vi "RageEquipCal_Lookup.vi"(0 "Record(abs path)":path=path "C:/SynologyDrive/ RaGE Systems/Test Equipment Cal Record/Rage_TestEquipmentCal.csv", 5 "SN / Active(1=T)":string[][](array[string])=[["MY53271104", "1"], ["MY57470396", "1"], ["MY48180752", "1"]], 11 "error in (no error)":errorcluster, 12 "Use Popup Warning(T)":bool=TRUE caption="Use Popup (T)", 13 "Run Vi (T)":bool=TRUE, 14 "Use Popup Warning(T)":bool caption="Check All SN's On List (T)") -> (4 "Status Summary Out":string[][](array[string]), 6 "OK":bool=TRUE, 15 "error out":errorcluster)   [LabVIEW 2018]
uses:
  Initialize References/Sequence Globals.vi
  <vilib>/Utility/file.llb/Read Delimited Spreadsheet (string).vi
  <vilib>/Utility/file.llb/Write Delimited Spreadsheet (string).vi
panel:
  out "RecordTempPath":path
  out "tmp path":path
  out "Mfr":string="RGA21-0197"
  out "Mfr_Index":i32
  out "Remind_Index":i32
  out "Active_index":i32[](array[numeric])=[11, 13, 14]
  out "ActiveList":string[][](array[string])
  out "RecordTempPath(str)":string="C:\\SynologyDrive\\ RaGE Systems\\Test Equipment Cal Record\\Rage_TestEquipmentCal.csv"
  out "HeaderMatchNames":string[](array[string])=["Model", "Last Cal Date", "SN", "Cal Due Date", "Desc", "Asset"]
  out "Header Match?":bool=TRUE
  out "expired?":bool=TRUE
  out "warn?":bool=TRUE
  out "Now":timestamp=timestamp(3806421519 s since 1904-01-01)
  out "Warn_Date":timestamp=timestamp(3776216400 s since 1904-01-01)
  out "seconds":dbl=2592000.0
  out "Warn (days)":string="30"
  out "last_cal(date)":timestamp=timestamp(3778808400 s since 1904-01-01)
  out "next_cal(date)":timestamp=timestamp(3778808400 s since 1904-01-01)
  out "asset":string="RGA21-0197"
  out "Asset_Index":i32
  out "desc":string="SIGGEN"
  out "Desc_Index":i32=6
  out "sn":string="MY48180752"
  out "next_cal(str)":string="9/29/2023"
  out "last_cal(str)":string="9/29/2020"
  out "model":string="N5182A"
  out "SnMatch?":bool=TRUE
  out "data_rows":string[][](array[string])=[["", "", "Anritsu", "37369C", "Yes", "", "VNA", "REPAIR(LOW)?", "", "", "E15539", "1/1/2001", "1/1/2001", "", "N/A", "N/A"], ["", "12989", "AstroAI", "DM6000AR", "Yes", "", "DMM", "LOWELL", "RaGE Systems", "", "2125220590", "1/1/2001", "1/1/2001", "", "N/A", "N/A"], ["", "12990", "AstroAI", "DM6000AR", "Yes", "", "DMM", "LOWELL", "RaGE Systems", "", "2125219987", "1/1/2001", "1/1/2001", "", "N/A", "N/A"], ["RGA20-0121", "", "Keithly", "2000", "Yes", "LAB-DC", "DMM", "LOWELL", "RaGE Systems", "Purchased", "727501", "1/1/2001", "1/1/2001", "", "N/A", "N/A"], ["RGA20-0123", "", "Keithly", "2000", "Yes", "LAB-DC", "DMM", "LOWELL", "RaGE Systems", "Purchased", "822794", "1/1/2001", "1/1/2001", "", "N/A", "N/A"], ["", "12937", "Keithly", "2000", "Yes", "Keithley 2000 Multimeters ", "DMM", "LOWELL", "RaGE Systems", "", "735571", "9/25/2019", "9/25/2020", "", "N/A", "N/A"], ["", "13071", "Keithly", "2700", "No", "LAB-DC", "DAQ", "LOWELL", "RaGE Systems", "", "", "Cal Not Required", "Cal Not Required", "", "N/A", "N/A"], ["RGA19-0071", "12928", "Keysight", "E5052A", "Yes", "LAB-RF", "Signal Source Analyzer", "LOWELL", "RaGE Systems (PRF)", "PRF", "MY44200746", "1/1/2001", "1/1/2001", "", "N/A", "N/A"], ["RGA19-0078", "12944", "Keysight", "8720ES", "Yes", "LAB-RF", "VNA", "LOWELL", "RaGE Systems", "Ks MVO -ebay", "US39173304", "8/28/2017", "8/28/2018", "F-Support  ", "N/A", "N/A"], ["RGA20-0130", "", "Keysight", "U2022XA", "Yes", "LAB-RF", "Power Meter", "WAM-PROD", "RaGE Systems", "Keysight", "MY58240013", "6/19/2018", "6/19/2020", "F-Support  ", "N/A", "TBD"], ["RGA20-0150", "", "Keysight", "N4692A", "Yes", "LAB-RF", "E-Cal Module", "WAM-PROD", "RaGE Systems", "Purchased", "MY62230410", "9/18/2019", "9/18/2021", "T", "N/A", "N/A"], ["RGA21-0195", "", "Keysight", "N5173B", "Yes", "LAB-RF", "Signal Generator", "WAM ATE-2", "RaGE Systems", "Purchased", "MY53271104", "11/6/2019", "11/6/2022", "T", "N/A", "1/19/2020"], ["RGA21-0224", "", "Keysight", "N5232B ", "Yes", "LAB-RF", "PNA", "WAM ATE-2", "RaGE Systems", "Purchased", "MY52221531", "2/20/2020", "2/20/2022", "T", "N/A", "N/A"], ["RGA21-0226", "", "Keysight", "N9010B", "No", "LAB-RF", "Spectrum Analyzer", "WAM ATE-2", "RaGE Systems", "Purchased", "MY57470396", "9/30/2023", "9/30/2025", "T", "N/A", "4/10/2025"], ["RGA21-0197", "12943", "Keysight", "N5182A", "Yes", "LAB-RF", "SIGGEN", "LOWELL", "RaGE Systems", "Purchased", "MY48180752", "9/29/2020", "9/29/2023", "T", "11/30/2024", "11/30/2023"], ["RGA21-0196", "", "Keysight", "N9010B", "Yes", "LAB-RF", "Spectrum Analyzer", "KS REPAIR", "RaGE Systems", "Purchased", "MY57110230", "11/3/2021", "11/3/2023", "T", "7/23/2024", "7/23/2024"], ["RGA21-0223", "12941", "Keysight", "N9020A", "Yes", "LAB-RF", "Spectrum Analyzer", "LOWELL", "Interlligent (Rental)", "Rent2Own", "MY49100234", "4/8/2021", "4/8/2023", "T", "N/A", "N/A"], ["RGA21-0222", "", "Keysight", "N5173B", "Yes", "LAB-RF", "SIGGEN", "WAM ATE-1", "RaGE Systems", "Purchased", "MY53270534 ", "6/12/2020", "6/12/2023", "T", "7/19/2020", "1/19/2021"], ["RGA21-0225", "", "Keysight", "N5232A", "Yes", "LAB-RF", "PNA", "WAM ATE-1", "RaGE Systems", "Purchased", "US52120122", "4/21/2021", "4/21/2023", "T", "6/6/2019", "6/8/2019"], ["RGA20-0149", "12945", "Keysight", "N5224B", "Yes", "LAB-RF", "PNA-X", "NBPT", "RaGE Systems", "Purchased", "MY55441806", "11/19/2019", "11/19/2021", "T", "2/11/2026", "2/11/2026"], ["N/A", "", "Keysight", "E4447A", "Yes", "LAB-RF", "Spectrum Analyzer", "WAM ATE-1", "LEIDOS", "Loaner", "MY9420095", "1/1/2001", "1/1/2001", "F  ", "N/A", "N/A"], ["RGA18-0064", "12942", "Keysight / Agilent", "E4433B", "Yes", "LAB-RF", "Signal Generator", "LOWELL", "RaGE Systems", "Ebay", "US40051660", "TBD", "TBD", "F-Support", "", ""], ["RGA18-0006", "12935", "Keysight / Agilent", "34401A", "Yes", "LAB-DC", "DMM", "LOWELL", "RaGE Systems", "Ebay", "MY44006486", "TBD", "TBD", "F-Support", "", ""], ["RGA18-0065", "12914", "Keysight / HP", "E4405B", "Yes", "LAB-RF", "Spectrum Analyzer", "LOWELL", "RaGE Systems", "Ebay", "US39440417", "TBD", "TBD", "F-Support", "", ""], ["RGA19-0072", "", "MINI - CIRCUITS", "PWR-6GHS", "Yes", "LAB-RF", "Power Meter", "LOWELL", "RaGE Systems", "PRF", "11807080018", "TBD", "TBD", "", "", ""], ["RGA19-0088", "", "National Instruments", "USB-TC01", "No", "LAB-Test", "Thermocouple", "LOWELL", "RaGE Systems", "Purchased", "N/A", "N/A", "N/A", "", "", ""], ["RGA18-0057", "13072", "Omega", "TCIC", "No", "LAB-Test", "Thermocouple", "LOWELL", "RaGE Systems", "Purchased", "N/A", "N/A", "N/A", "", "", ""], ["RGA20-0104", "", "Vaunix", "LPS-802", "No", "LAB-Test", "Vaunix Lab Brick LPS-802 4 – 8 GHz USB Programmable Phase Shifter", "LOWELL", "RaGE Systems", "Purchased", "N/A", "N/A", "N/A", "", "", ""], ["RGA20-0105", "12900", "Vaunix", "LDA-602", "No", "LAB-Test", "Vaunix Lab Brick Digital Attenuator LDA-602", "LOWELL", "RaGE Systems", "Purchased", "N/A", "N/A", "N/A", "", "", ""]]
  out "SN_Index":i32=10
  out "Model_Index":i32=3
  out "NextCal_Index":i32=12
  out "LastCal_Index":i32=11
  out "Record(ary)":string[][](array[string])=[["Asset", "Security Label Number", "Manufacturer", "Model", "Calibration Required (Yes/No)", "Type", "Desc", "Location or User", "Owner / Loan", "Provided By", "SN", "Last Cal Date", "Cal Due Date", "Keysight Asseted", "Keysight Cal Entitlement Expires", "Keysight Warranty Expires"], ["", "", "Anritsu", "37369C", "Yes", "", "VNA", "REPAIR(LOW)?", "", "", "E15539", "1/1/2001", "1/1/2001", "", "N/A", "N/A"], ["", "12989", "AstroAI", "DM6000AR", "Yes", "", "DMM", "LOWELL", "RaGE Systems", "", "2125220590", "1/1/2001", "1/1/2001", "", "N/A", "N/A"], ["", "12990", "AstroAI", "DM6000AR", "Yes", "", "DMM", "LOWELL", "RaGE Systems", "", "2125219987", "1/1/2001", "1/1/2001", "", "N/A", "N/A"], ["RGA20-0121", "", "Keithly", "2000", "Yes", "LAB-DC", "DMM", "LOWELL", "RaGE Systems", "Purchased", "727501", "1/1/2001", "1/1/2001", "", "N/A", "N/A"], ["RGA20-0123", "", "Keithly", "2000", "Yes", "LAB-DC", "DMM", "LOWELL", "RaGE Systems", "Purchased", "822794", "1/1/2001", "1/1/2001", "", "N/A", "N/A"], ["", "12937", "Keithly", "2000", "Yes", "Keithley 2000 Multimeters ", "DMM", "LOWELL", "RaGE Systems", "", "735571", "9/25/2019", "9/25/2020", "", "N/A", "N/A"], ["", "13071", "Keithly", "2700", "No", "LAB-DC", "DAQ", "LOWELL", "RaGE Systems", "", "", "Cal Not Required", "Cal Not Required", "", "N/A", "N/A"], ["RGA19-0071", "12928", "Keysight", "E5052A", "Yes", "LAB-RF", "Signal Source Analyzer", "LOWELL", "RaGE Systems (PRF)", "PRF", "MY44200746", "1/1/2001", "1/1/2001", "", "N/A", "N/A"], ["RGA19-0078", "12944", "Keysight", "8720ES", "Yes", "LAB-RF", "VNA", "LOWELL", "RaGE Systems", "Ks MVO -ebay", "US39173304", "8/28/2017", "8/28/2018", "F-Support  ", "N/A", "N/A"], ["RGA20-0130", "", "Keysight", "U2022XA", "Yes", "LAB-RF", "Power Meter", "WAM-PROD", "RaGE Systems", "Keysight", "MY58240013", "6/19/2018", "6/19/2020", "F-Support  ", "N/A", "TBD"], ["RGA20-0150", "", "Keysight", "N4692A", "Yes", "LAB-RF", "E-Cal Module", "WAM-PROD", "RaGE Systems", "Purchased", "MY62230410", "9/18/2019", "9/18/2021", "T", "N/A", "N/A"], ["RGA21-0195", "", "Keysight", "N5173B", "Yes", "LAB-RF", "Signal Generator", "WAM ATE-2", "RaGE Systems", "Purchased", "MY53271104", "11/6/2019", "11/6/2022", "T", "N/A", "1/19/2020"], ["RGA21-0224", "", "Keysight", "N5232B ", "Yes", "LAB-RF", "PNA", "WAM ATE-2", "RaGE Systems", "Purchased", "MY52221531", "2/20/2020", "2/20/2022", "T", "N/A", "N/A"], ["RGA21-0226", "", "Keysight", "N9010B", "No", "LAB-RF", "Spectrum Analyzer", "WAM ATE-2", "RaGE Systems", "Purchased", "MY57470396", "9/30/2023", "9/30/2025", "T", "N/A", "4/10/2025"], ["RGA21-0197", "12943", "Keysight", "N5182A", "Yes", "LAB-RF", "SIGGEN", "LOWELL", "RaGE Systems", "Purchased", "MY48180752", "9/29/2020", "9/29/2023", "T", "11/30/2024", "11/30/2023"], ["RGA21-0196", "", "Keysight", "N9010B", "Yes", "LAB-RF", "Spectrum Analyzer", "KS REPAIR", "RaGE Systems", "Purchased", "MY57110230", "11/3/2021", "11/3/2023", "T", "7/23/2024", "7/23/2024"], ["RGA21-0223", "12941", "Keysight", "N9020A", "Yes", "LAB-RF", "Spectrum Analyzer", "LOWELL", "Interlligent (Rental)", "Rent2Own", "MY49100234", "4/8/2021", "4/8/2023", "T", "N/A", "N/A"], ["RGA21-0222", "", "Keysight", "N5173B", "Yes", "LAB-RF", "SIGGEN", "WAM ATE-1", "RaGE Systems", "Purchased", "MY53270534 ", "6/12/2020", "6/12/2023", "T", "7/19/2020", "1/19/2021"], ["RGA21-0225", "", "Keysight", "N5232A", "Yes", "LAB-RF", "PNA", "WAM ATE-1", "RaGE Systems", "Purchased", "US52120122", "4/21/2021", "4/21/2023", "T", "6/6/2019", "6/8/2019"], ["RGA20-0149", "12945", "Keysight", "N5224B", "Yes", "LAB-RF", "PNA-X", "NBPT", "RaGE Systems", "Purchased", "MY55441806", "11/19/2019", "11/19/2021", "T", "2/11/2026", "2/11/2026"], ["N/A", "", "Keysight", "E4447A", "Yes", "LAB-RF", "Spectrum Analyzer", "WAM ATE-1", "LEIDOS", "Loaner", "MY9420095", "1/1/2001", "1/1/2001", "F  ", "N/A", "N/A"], ["RGA18-0064", "12942", "Keysight / Agilent", "E4433B", "Yes", "LAB-RF", "Signal Generator", "LOWELL", "RaGE Systems", "Ebay", "US40051660", "TBD", "TBD", "F-Support", "", ""], ["RGA18-0006", "12935", "Keysight / Agilent", "34401A", "Yes", "LAB-DC", "DMM", "LOWELL", "RaGE Systems", "Ebay", "MY44006486", "TBD", "TBD", "F-Support", "", ""], ["RGA18-0065", "12914", "Keysight / HP", "E4405B", "Yes", "LAB-RF", "Spectrum Analyzer", "LOWELL", "RaGE Systems", "Ebay", "US39440417", "TBD", "TBD", "F-Support", "", ""], ["RGA19-0072", "", "MINI - CIRCUITS", "PWR-6GHS", "Yes", "LAB-RF", "Power Meter", "LOWELL", "RaGE Systems", "PRF", "11807080018", "TBD", "TBD", "", "", ""], ["RGA19-0088", "", "National Instruments", "USB-TC01", "No", "LAB-Test", "Thermocouple", "LOWELL", "RaGE Systems", "Purchased", "N/A", "N/A", "N/A", "", "", ""], ["RGA18-0057", "13072", "Omega", "TCIC", "No", "LAB-Test", "Thermocouple", "LOWELL", "RaGE Systems", "Purchased", "N/A", "N/A", "N/A", "", "", ""], ["RGA20-0104", "", "Vaunix", "LPS-802", "No", "LAB-Test", "Vaunix Lab Brick LPS-802 4 – 8 GHz USB Programmable Phase Shifter", "LOWELL", "RaGE Systems", "Purchased", "N/A", "N/A", "N/A", "", "", ""], ["RGA20-0105", "12900", "Vaunix", "LDA-602", "No", "LAB-Test", "Vaunix Lab Brick Digital Attenuator LDA-602", "LOWELL", "RaGE Systems", "Purchased", "N/A", "N/A", "N/A", "", "", ""]]
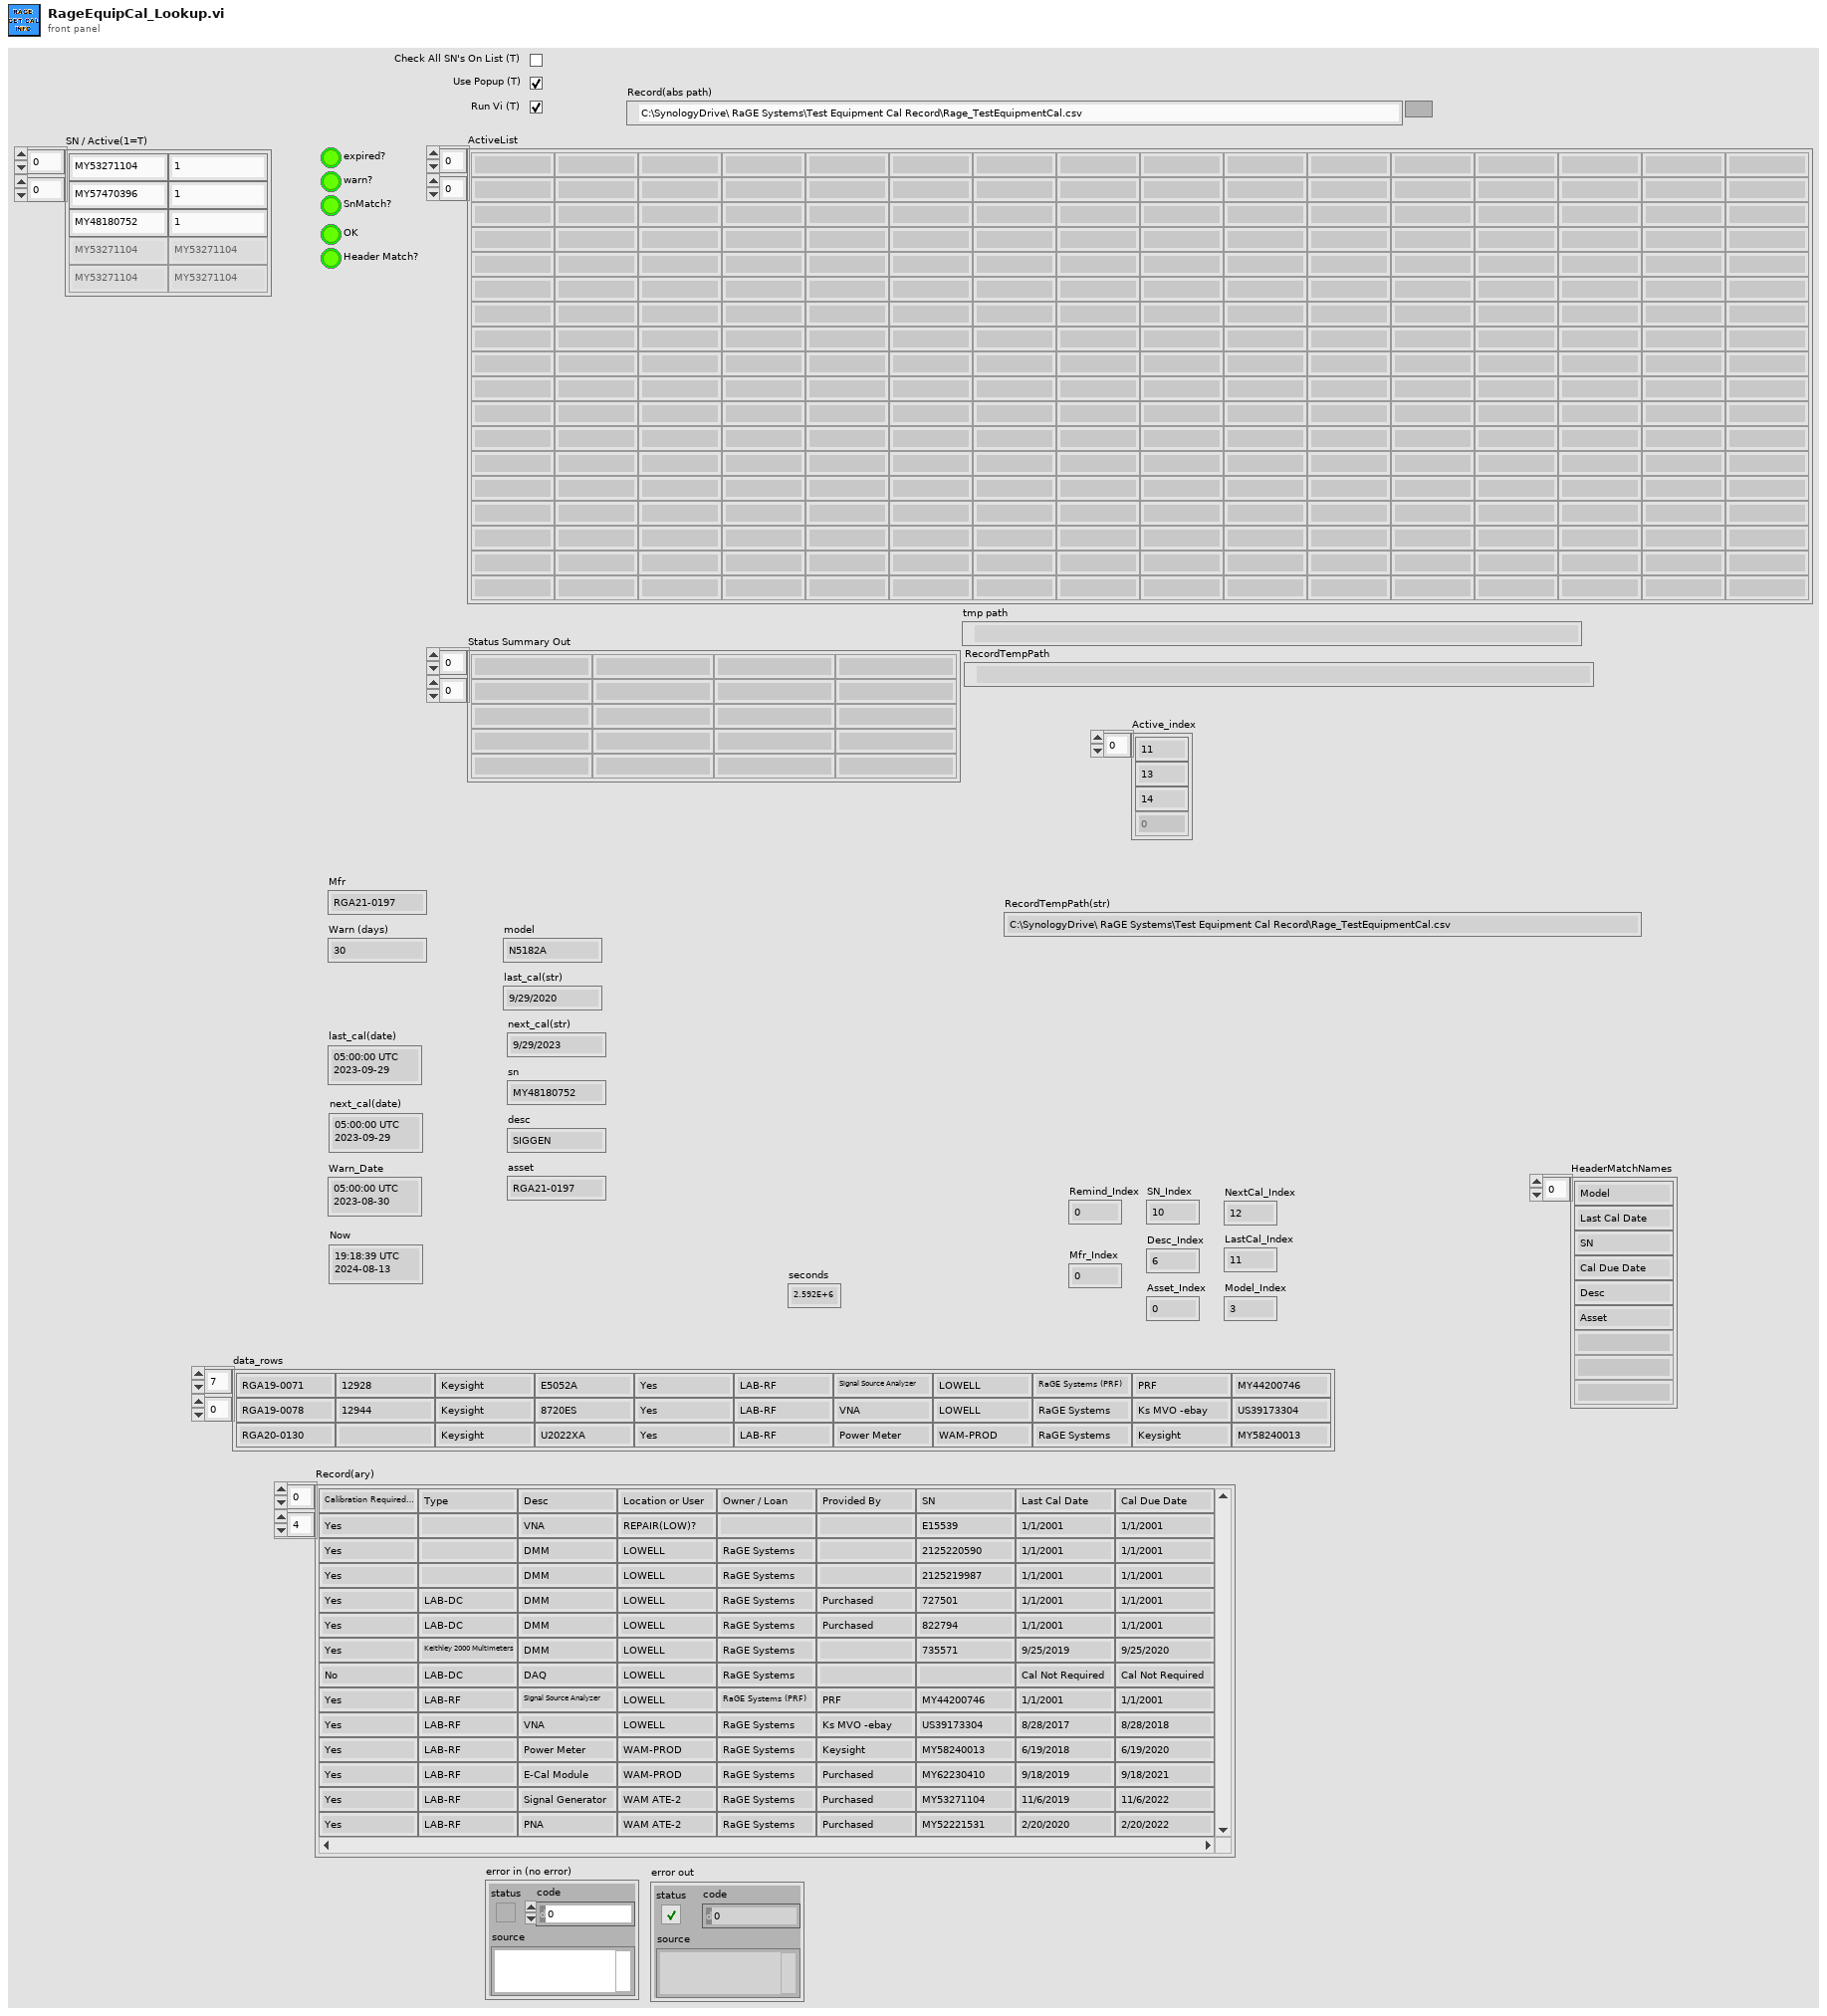
[diagram p1: front panel]
types:
  T1 = enum16{"Left Button", "Center Button", "Right Button", "Window Close"}
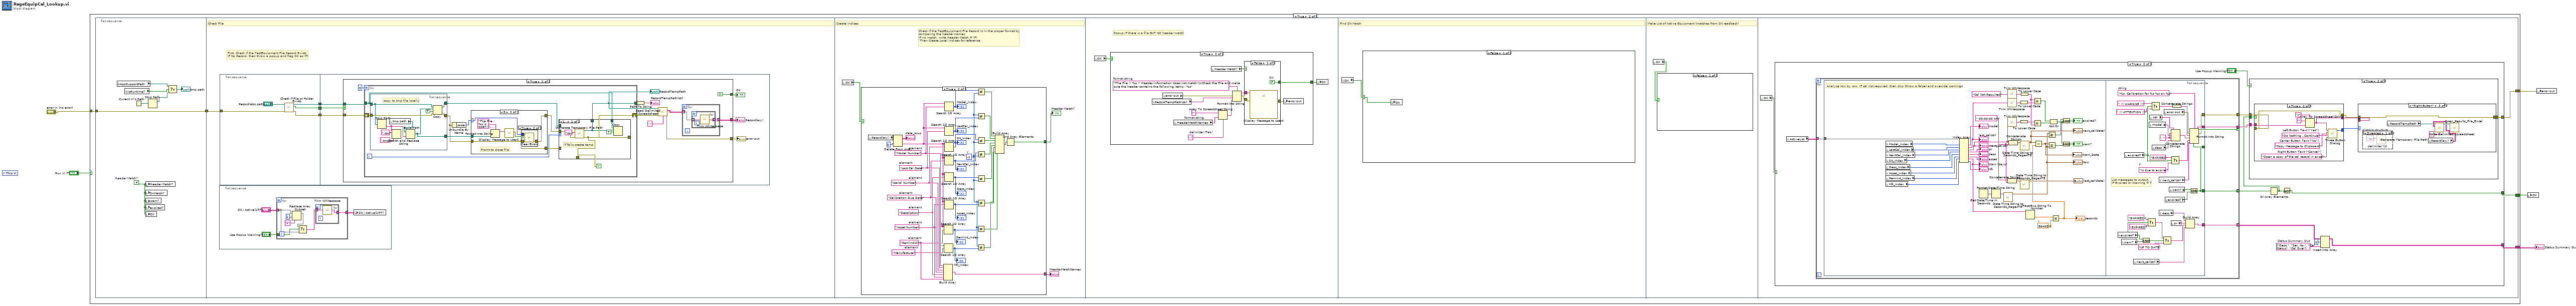
[diagram p0: block diagram]
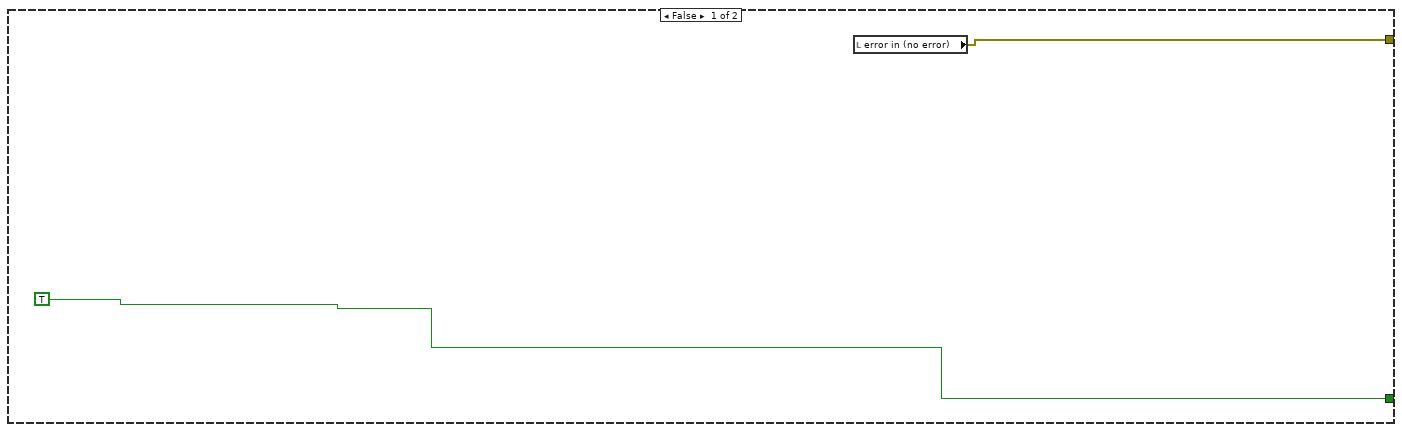
[diagram p2: hidden frame]
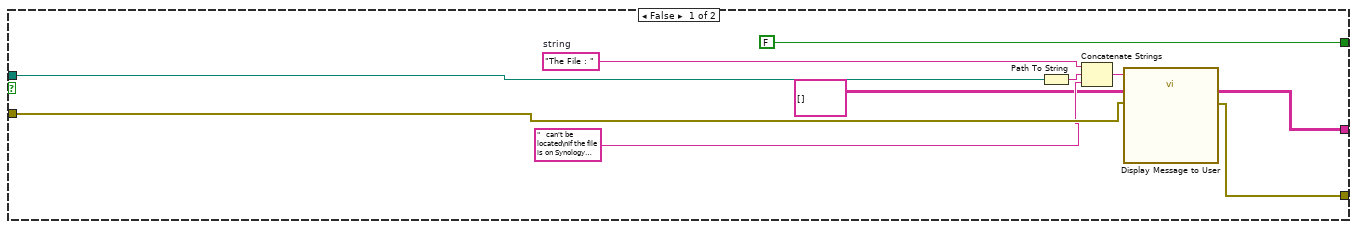
[diagram p3: hidden frame]
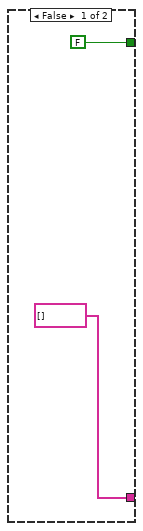
[diagram p7: hidden frame]
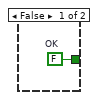
[diagram p8: hidden frame]
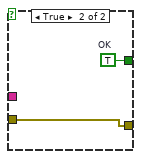
[diagram p9: hidden frame]
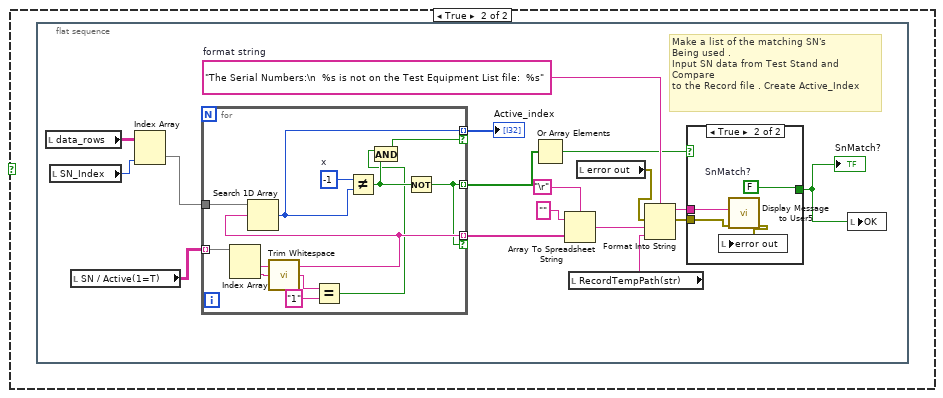
[diagram p10: hidden frame]
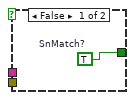
[diagram p11: hidden frame]
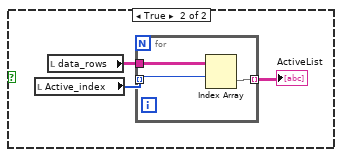
[diagram p12: hidden frame]
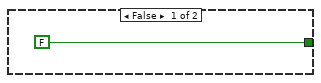
[diagram p13: hidden frame]
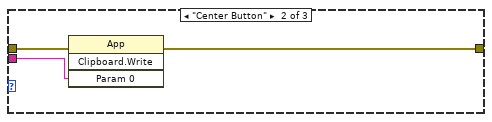
[diagram p16: hidden frame]
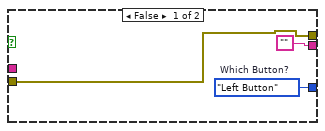
[diagram p18: hidden frame]
diagram:
  n1 = control-ref of="This VI"() -> ()  [unwired: 1 out]
  n2 = case shown="True" "Run Vi (T)" {
    tunnel: "error in (no error)" -> [_ w12]
    tunnel: [w7 w11] -> w4
    tunnel: [TRUE w10] -> w2
    tunnel: [_ w9] -> w1
    frame False {
      n3 = local read "error in (no error)"() -> (w7:errorcluster)
    }
    frame True {
      n4 = flat-sequence {
        tunnel: w12 -> [w19]
        tunnel: [w19] -> w8
        tunnel: w8 -> [w20]
        tunnel: [w218] -> w11
        tunnel: [w217] -> w10
        tunnel: [w216] -> w9
        frame #0 {
          w18 = FALSE  # Header Match?
          n5 = global read "Sequence Globals.vi" "AppSupportPath"() -> (w16:path)
          n6 = global read "Sequence Globals.vi" "IsRuntime?"() -> (w17:bool)
          n7 = Current VI's Path() -> (path=w15:path)
          n8 = local write "Header Match?"(w18) -> ()
          n9 = local write "SnMatch?"(w18) -> ()
          n10 = local write "warn?"(w18) -> ()
          n11 = local write "expired?"(w18) -> ()
          n12 = local write "OK"(w18) -> ()
          n13 = Strip Path(path=w15) -> (stripped path=w14:path)  [unwired: 1 out]
          n14 = Select(t=w16, s=w17, f=w14) -> (s? t:f=→"tmp path":path)
        }
        frame #1 {
          # "First, Check If the TestEquipment File Record Exists\nIF No Record, then throw a popup and flag OK as (F)"
          # "Check File"
          n15 = flat-sequence {
            frame #0 {
              n16 = for {
                tunnel: "SN / Active(1=T)" -> [w30] mode=indexing
                tunnel: [w33] -> w25 mode=indexing
                tunnel: "Use Popup Warning(T)" -> [w27]
                n17 = Replace Array Subset(array=w30, new element="1" ("new element/subarray"), index=1) -> (w28:string[])
                n18 = Select(t=w28, s=w27, f=w30) -> (s? t:f=w29:string[])
                n19 = for {
                  tunnel: w29 -> [w35] mode=indexing
                  tunnel: [w34] -> w33 mode=indexing
                  n20 = call <vilib>:"Trim Whitespace.vi"("string"=w35) -> ("trimmed string"=w34:string)  [unwired: 1 in]
                }
              }
              n21 = local write "SN / Active(1=T)"(w25) -> ()
            }
          }
          n22 = flat-sequence {
            tunnel: [w39] -> w23
            tunnel: [w40] -> w22
            tunnel: [w38] -> w21
            tunnel: w20 -> [w37]
            tunnel: w23 -> [w46]
            tunnel: w22 -> [w45]
            tunnel: w21 -> [w44]
            frame #0 {
              n23 = call <vilib>:"Check if File or Folder Exists.vi"("error in (no error)"=w37, "path"="Record(abs path)") -> ("error out"=w40:errorcluster, "file or folder exists?"=w39:bool, "dup path"=w38:path)  [unwired: 7 in]
            }
            frame #1 {
              n24 = case shown="True" w46 {
                tunnel: w45 -> [w50 w62]
                tunnel: w44 -> [w55 w63]
                tunnel: [FALSE TRUE] -> w43
                tunnel: [w49 w60] -> w42
                tunnel: [string[][] [] w64] -> w41
                frame False {
                  w53 = "The File : "  # string
                  n25 = Path To String(path=w55) -> (string=w54:string)
                  n26 = Concatenate Strings(w53, w54, "   can't be located\nIf the file is on Synology Drive check the connection to the server" ("string")) -> (w52:string)
                  n27 = call "Display Message to User"("error in (no error)"=w50, "Message"=w52) -> ("error out"=w49:errorcluster)  [unwired: 8 in, 1 out]
                }
                frame True {
                  n28 = for {
                    N: 3 -> [_]
                    shift-right: [w71] -> w58
                    shift-left: w62 -> [w78]
                    tunnel: w63 -> [w67]
                    tunnel: [w72] -> w57
                    i -> [w75]
                    stop <- w69 continue-if-true
                    n29 = flat-sequence {
                      tunnel: w67 -> [w102]
                      tunnel: w78 -> [w108]
                      tunnel: [w107] -> w70
                      tunnel: [w106] -> w73
                      tunnel: [w100] -> w76
                      frame #0 {
                        # "copy to tmp file locally"
                        n30 = Strip Path(path=w102) -> (name=w101:string)  [unwired: 1 out]
                        n31 = local read "tmp path"() -> (w103:path)
                        n32 = Search and Replace String(input string=w101, search string=".csv", replace string=".tmp" ("replace string (\"\")")) -> ()  [unwired: 5 in, 4 out]
                        n33 = Build Path(base path=w103, name or relative path=w101) -> (appended path=w100:path)
                        n34 = Copy(8:w108, 9:TRUE ("overwrite (F)"), 10:w100, 11:w102) -> (0:w107:errorcluster, 3:w106:path)  [unwired: 1 in, 1 out]
                      }
                    }
                    n35 = Unbundle By Name(w70) -> ("code"=w77:i32)
                    n36 = case shown="5" w77 {
                      selector: w77 -> [_ w91]
                      tunnel: [w88 w93] -> w74
                      tunnel: w70 -> [w88 w89]
                      tunnel: w76 -> [_ w92]
                      tunnel: [w88 w89] -> w68
                      frame 0, Default {
                      }
                      frame 5 {
                        # "Promt to close file"
                        n37 = Format Into String(format string="The File : %s is open!! \nClose the file and press OK to continue", w92) -> (resulting string=w94:string)  [unwired: 2 in, 1 out]
                        n38 = call "Display Message to User2"("Message"=w94) -> ("OK"=w90:bool)  [unwired: 9 in, 1 out]
                        n39 = case shown="True" w90 {
                          tunnel: [w96 w99] -> w93
                          tunnel: w91 -> [_ w98]
                          tunnel: w89 -> [w96 w97]
                          frame False {
                          }
                          frame True {
                            n40 = call <vilib>:"Clear Errors.vi"("error in (no error)"=w97, "specific error code to clear (0: all)"=w98) -> ("error out"=w99:errorcluster)  [unwired: 4 in, 1 out]
                          }
                        }
                      }
                    }
                    n41 = case shown="2.." w75 {
                      tunnel: w74 -> [w80 w87]
                      tunnel: w73 -> [w81 _]
                      tunnel: [w81 w85] -> w72
                      tunnel: [w80 w86] -> w71
                      tunnel: [w79 w86] -> w69
                      tunnel: w68 -> [w79 _]
                      tunnel: w67 -> [_ w84]
                      frame 0, Default {
                      }
                      frame 2.. {
                        # "If fails create temp"
                        n42 = call <vilib>:"Generate Temporary File Path.vi"("error in (no error)"=w87, "Temporary File Extension (tmp)"="csv") -> ("error out"=w86:errorcluster, "Unique Temporary File Path"=w85:path)  [unwired: 8 in]
                        n43 = Copy(9:TRUE ("overwrite (F)"), 10:w85, 11:w84) -> ()  [unwired: 2 in, 3 out]
                      }
                    }
                  }
                  "RecordTempPath" <- w57
                  n44 = Path To String(path=w57) -> (string=→"RecordTempPath(str)":string)
                  n45 = call-poly <vilib>:"Read Delimited Spreadsheet.vi"("file path (dialog if empty)"=w57, "error in (no error)"=w58, "delimiter (\\t)"="," ("delimiter (\\t)")) -> ("all rows"=w61:string[][], "error out"=w60:errorcluster)  [unwired: 7 in, 4 out]
                  n46 = for {
                    tunnel: w61 -> [w111] mode=indexing
                    tunnel: [w110] -> w64 mode=indexing
                    n47 = for {
                      tunnel: w111 -> [w113] mode=indexing
                      tunnel: [w112] -> w110 mode=indexing
                      n48 = call <vilib>:"Trim Whitespace.vi"("string"=w113) -> ("trimmed string"=w112:string)  [unwired: 1 in]
                    }
                  }
                }
              }
              "OK" <- w43
              "error out" <- w42
              "Record(ary)" <- w41
            }
          }
        }
        frame #2 {
          # "Check If the TestEquipment File Record Is in the proper format by\ncomparing the header names.\nIF no match, write Header Match = (F)\n Then Create Local indices for reference"
          # "Create indices"
          n49 = local read "OK"() -> (w114:bool)
          n50 = case shown="True" w114 {
            tunnel: [string[] [] w129] -> w116
            tunnel: [FALSE w127] -> w115
            frame False {
            }
            frame True {
              w119 = "Manufacturer"  # element
              w125 = "Remind(d)"  # element
              w130 = "Asset Number"  # element
              w131 = "Description"  # element
              w121 = -1  # y
              w133 = "Serial Number"  # element
              w135 = "Model Number"  # element
              w132 = "Calibration Due Date"  # element
              w134 = "Last Cal Date"  # element
              n51 = local read "Record(ary)"() -> (w150:string[][])
              n52 = Delete From Array(array=w150, index (row)=0) -> (deleted portion=w120:string[], array with subset deleted=→"data_rows":string[][])  [unwired: 2 in]
              n53 = Build Array(w135, w134, w133, w132, w131, w130, w125) -> (w129:string[])
              n54 = Search 1D Array(1D array=w120, element=w125) -> (index of element=w126:i32)  [unwired: 1 in]
              "Remind_Index" <- w126
              n55 = Search 1D Array(1D array=w120, element=w119) -> (index of element=w123:i32)  [unwired: 1 in]
              "Mfr_Index" <- w123
              n56 = Search 1D Array(1D array=w120, element=w135) -> (index of element=w147:i32)  [unwired: 1 in]
              "Model_Index" <- w147
              n57 = Search 1D Array(1D array=w120, element=w134) -> (index of element=w146:i32)  [unwired: 1 in]
              "LastCal_Index" <- w146
              n58 = Search 1D Array(1D array=w120, element=w133) -> (index of element=w145:i32)  [unwired: 1 in]
              "SN_Index" <- w145
              n59 = Search 1D Array(1D array=w120, element=w132) -> (index of element=w144:i32)  [unwired: 1 in]
              "NextCal_Index" <- w144
              n60 = Search 1D Array(1D array=w120, element=w131) -> (index of element=w143:i32)  [unwired: 1 in]
              "Desc_Index" <- w143
              n61 = Search 1D Array(1D array=w120, element=w130) -> (index of element=w142:i32)  [unwired: 1 in]
              "Asset_Index" <- w142
              n62 = Not Equal?(x=w121, y=w126) -> (x != y?=w124:bool)
              n63 = Not Equal?(x=w121, y=w123) -> (x != y?=w122:bool)
              n64 = Not Equal?(x=w147, y=w121) -> (x != y?=w141:bool)
              n65 = Not Equal?(x=w121, y=w146) -> (x != y?=w140:bool)
              n66 = Not Equal?(x=w145, y=w121) -> (x != y?=w139:bool)
              n67 = Not Equal?(x=w144, y=w121) -> (x != y?=w138:bool)
              n68 = Not Equal?(x=w143, y=w121) -> (x != y?=w137:bool)
              n69 = Not Equal?(x=w121, y=w142) -> (x != y?=w136:bool)
              n70 = Build Array(w141, w140, w139, w138, w137, w136, w124, w122) -> (w128:bool[])
              n71 = And Array Elements(Boolean array=w128) -> (logical AND=w127:bool)
            }
          }
          "Header Match?" <- w115
          "HeaderMatchNames" <- w116
        }
        frame #3 {
          # "Popup IF there is a file BUT NO header match"
          n72 = local read "OK"() -> (w152:bool)
          n73 = case shown="True" w152 {
            tunnel: [w153 w154] -> w151
            frame False {
              w153 = FALSE  # OK
            }
            frame True {
              w158 = ""  # format string
              w160 = ","  # delimiter (Tab)
              w163 = "The File < %s > Header information does not match!!\nCheck the File and make sure the header contains the following items : %s"  # format string
              n74 = local read "RecordTempPath(str)"() -> (w165:string)
              n75 = local read "error out"() -> (w157:errorcluster)
              n76 = local read "HeaderMatchNames"() -> (w161:string[])
              n77 = local read "Header Match?"() -> (w159:bool)
              n78 = Array To Spreadsheet String(delimiter (Tab)=w160, array=w161, 3:w158) -> (spreadsheet string=w162:string)
              n79 = Format Into String(format string=w163, error in=w157, w165, w162) -> (resulting string=w164:string, error out=w156:errorcluster)  [unwired: 1 in]
              n80 = case shown="False" w159 {
                tunnel: w164 -> [w169 _]
                tunnel: w156 -> [w168 w171]
                tunnel: [w167 w171] -> w155
                tunnel: [w166 w170] -> w154
                frame False {
                  w166 = FALSE  # OK
                  n81 = call "Display Message to User4"("error in (no error)"=w168, "Message"=w169) -> ("error out"=w167:errorcluster)  [unwired: 8 in, 1 out]
                }
                frame True {
                  w170 = TRUE  # OK
                }
              }
              n82 = local write "error out"(w155) -> ()
            }
          }
          n83 = local write "OK"(w151) -> ()
        }
        frame #4 {
          # "Find SN Match"
          n84 = local read "OK"() -> (w172:bool)
          n85 = case shown="False" w172 {
            selector: w172 -> [w173 _]
            frame False {
              n86 = local write "OK"(w173) -> ()
            }
            frame True {
              n87 = flat-sequence {
                frame #0 {
                  w187 = "The Serial Numbers:\n  %s is not on the Test Equipment List file:  %s"  # format string
                  # "Make a list of the matching SN's\nBeing used . \nInput SN data from Test Stand and Compare\nto the Record file . Create Active_Index"
                  n88 = local read "data_rows"() -> (w188:string[][])
                  n89 = local read "SN_Index"() -> (w190:i32)
                  n90 = local read "SN / Active(1=T)"() -> (w174:string[][])
                  n91 = Index Array(array=w188, index (col)=w190) -> (element=w189:string[])  [unwired: 1 in]
                  n92 = for {
                    tunnel: w189 -> [w207]
                    tunnel: [w202] -> w185 mode=indexing if=w198
                    tunnel: w174 -> [w203] mode=indexing
                    tunnel: [w204] -> w179 mode=indexing if=w197
                    tunnel: [w198] -> w178 mode=indexing
                    w206 = -1  # x
                    n93 = Index Array(array=w203) -> (element #1=w202:string, element #2=w201:string)  [unwired: 2 in]
                    n94 = Search 1D Array(1D array=w207, element=w202) -> (index of element=w204:i32)  [unwired: 1 in]
                    n95 = call <vilib>:"Trim Whitespace.vi"("string"=w201) -> ("trimmed string"=w199:string)  [unwired: 1 in]
                    n96 = Equal?(x=w199, y="1") -> (x = y?=w196:bool)
                    n97 = Not Equal?(x=w206, y=w204) -> (x != y?=w205:bool)
                    n98 = And(x=w196, y=w205) -> (x .and. y?=w197:bool)
                    n99 = Not(x=w205) -> (.not. x?=w198:bool)
                  }
                  "Active_index" <- w179
                  n100 = Or Array Elements(Boolean array=w178) -> (logical OR=w181:bool)
                  n101 = Array To Spreadsheet String(delimiter (Tab)="\r", array=w185, 3:"" ("format string")) -> (spreadsheet string=w186:string)
                  n102 = local read "RecordTempPath(str)"() -> (w183:string)
                  n103 = local read "error out"() -> (w176:errorcluster)
                  n104 = Format Into String(format string=w187, error in=w176, w186, w183) -> (resulting string=w182:string, error out=w175:errorcluster)  [unwired: 1 in]
                  n105 = case shown="True" w181 {
                    tunnel: w182 -> [_ w195]
                    tunnel: [w191 w194] -> w177
                    tunnel: w175 -> [_ w193]
                    frame False {
                      w191 = TRUE  # SnMatch?
                    }
                    frame True {
                      w194 = FALSE  # SnMatch?
                      n106 = call "Display Message to User5"("error in (no error)"=w193, "Message"=w195) -> ("error out"=w192:errorcluster)  [unwired: 8 in, 1 out]
                      n107 = local write "error out"(w192) -> ()
                    }
                  }
                  "SnMatch?" <- w177
                  n108 = local write "OK"(w177) -> ()
                }
              }
            }
          }
        }
        frame #5 {
          # "Make List of Active Equipment (matches from SN readback)"
          n109 = local read "OK"() -> (w208:bool)
          n110 = case shown="False" w208 {
            frame False {
            }
            frame True {
              n111 = local read "Active_index"() -> (w210:i32[])
              n112 = local read "data_rows"() -> (w211:string[][])
              n113 = for {
                tunnel: w211 -> [w214]
                tunnel: [w212] -> w209 mode=indexing
                tunnel: w210 -> [w213] mode=indexing
                n114 = Index Array(array=w214, index (row)=w213) -> (element=w212:string[])  [unwired: 1 in]
              }
              "ActiveList" <- w209
            }
          }
        }
        frame #6 {
          n115 = local read "OK"() -> (w215:bool)
          n116 = case shown="True" w215 {
            tunnel: [_ w223] -> w218
            tunnel: [FALSE w222] -> w217
            tunnel: [_ w221] -> w216
            frame False {
            }
            frame True {
              w227 = string[] ["Desc.", "Ser. No.", "Cal Status", "Cal Due"]  # Status Summary Out
              n117 = local read "ActiveList"() -> (w229:string[][])
              n118 = for {
                tunnel: [w267] -> w231 mode=indexing if=w265
                tunnel: w229 -> [w266] mode=indexing
                tunnel: [w264] -> w230 mode=indexing
                tunnel: [w263] -> w228 mode=indexing
                tunnel: [w262] -> w224
                n119 = flat-sequence {
                  tunnel: w266 -> [w299]
                  tunnel: [w332] -> w267
                  tunnel: [w329] -> w265
                  tunnel: [w329] -> w264
                  tunnel: [w315] -> w263
                  tunnel: [w311] -> w262
                  frame #0 {
                    w272 = 86400.0  # y
                    w307 = " 00:00:00 AM" ("string")
                    # "Analyze row by row, IF cal not required, then skip (throw a false) and override warnings"
                    n120 = local read "Model_Index"() -> (w298:i32)
                    n121 = local read "LastCal_Index"() -> (w297:i32)
                    n122 = local read "NextCal_Index"() -> (w296:i32)
                    n123 = local read "SN_Index"() -> (w295:i32)
                    n124 = local read "Desc_Index"() -> (w294:i32)
                    n125 = local read "Asset_Index"() -> (w293:i32)
                    n126 = local read "Remind_Index"() -> (w274:i32)
                    n127 = local read "Mfr_Index"() -> (w269:i32)
                    n128 = Index Array(array=w299, index #1=w298, index #2=w297, index #3=w296, index #4=w295, index #5=w294, index #6=w293, index #7=w274, index #8=w269) -> (element #1=→"model":string, element #2=w288:string, element #3=w287:string, element #4=→"sn":string, element #5=→"desc":string, element #6=→"asset":string, element #7=w270:string, element #8=→"Mfr":string)
                    "last_cal(str)" <- w288
                    "next_cal(str)" <- w287
                    "Warn (days)" <- w270
                    n129 = Get Date/Time In Seconds() -> (seconds since 1Jan1904=w306:timestamp)
                    n130 = Format Date/Time String(seconds (now)=w306) -> (date/time string=w305:string)  [unwired: 2 in]
                    n131 = call "Date Time String to Seconds_RageATE.vi"("Time/date(str)in"=w305) -> ("Timestamp from Date/Time String"=w302:timestamp)  [unwired: 8 in, 2 out]
                    "Now" <- w302
                    n132 = call <vilib>:"Trim Whitespace.vi"("string"="Cal Not Required") -> ("trimmed string"=w285:string)  [unwired: 1 in]
                    n133 = call <vilib>:"Trim Whitespace.vi"("string"=w288) -> ("trimmed string"=w283:string)  [unwired: 1 in]
                    n134 = call <vilib>:"Trim Whitespace.vi"("string"=w287) -> ("trimmed string"=w281:string)  [unwired: 1 in]
                    n135 = Concatenate Strings(w287, w307) -> (w308:string)
                    n136 = Concatenate Strings(w287, w307) -> (w310:string)
                    n137 = To Lower Case(string=w283) -> (all lower case string=w282:string)
                    n138 = To Lower Case(string=w281) -> (all lower case string=w280:string)
                    n139 = To Lower Case(string=w285) -> (all lower case string=w284:string)
                    n140 = call "Date Time String to Seconds_RageATE.vi"("Time/date(str)in"=w310) -> ("Timestamp from Date/Time String"=w301:timestamp)  [unwired: 8 in, 2 out]
                    "next_cal(date)" <- w301
                    n141 = call "Date Time String to Seconds_RageATE.vi"("Time/date(str)in"=w308) -> ("Timestamp from Date/Time String"=→"last_cal(date)":timestamp)  [unwired: 8 in, 2 out]
                    n142 = Fract/Exp String To Number(string=w270) -> (number=w273:dbl)  [unwired: 3 in, 1 out]
                    n143 = Equal?(x=w284, y=w282) -> (x = y?=w279:bool)
                    n144 = Equal?(x=w280, y=w284) -> (x = y?=w278:bool)
                    n145 = Greater Or Equal?(x=w302, y=w301) -> (x >= y?=w300:bool)
                    n146 = Not Or(1:w278, 2:w279) -> (0:w275:bool)
                    n147 = Multiply(x=w273, y=w272) -> (x*y=w271:dbl)
                    "seconds" <- w271
                    n148 = Subtract(x=w301, y=w271) -> (x-y=w304:timestamp)
                    "Warn_Date" <- w304
                    n149 = Less Or Equal?(x=w304, y=w302) -> (x <= y?=w303:bool)
                    n150 = And(x=w300, y=w275) -> (x .and. y?=→"expired?":bool)
                    n151 = And(x=w275, y=w303) -> (x .and. y?=→"warn?":bool)
                  }
                  frame #1 {
                    w325 = ", "
                    w335 = "Is due to expire "  # f
                    w333 = "%s  Calibration for %s %s on %s"  # string
                    # "List messages to output\nIF Expired or Warning = T"
                    n152 = local read "expired?"() -> (w318:bool)
                    n153 = local read "warn?"() -> (w322:bool)
                    n154 = local read "expired?"() -> (w340:bool)
                    n155 = local read "next_cal(str)"() -> (w316:string)
                    n156 = And(x=w318, y=w322) -> (x .and. y?=w321:bool)
                    n157 = Select(t="EXPIRED ", s=w318, f="EXPIRES ") -> (s? t:f=w319:string)
                    n158 = local read "model"() -> (w343:string)
                    n159 = local read "Mfr"() -> (w326:string)
                    n160 = Select(t=" !!! WARNING !!!", s=w340, f=" !!! ATTENTION !!!") -> (s? t:f=w339:string)
                    n161 = local read "desc"() -> (w327:string)
                    n162 = local read "next_cal(str)"() -> (w342:string)
                    n163 = local read "desc"() -> (w313:string)
                    n164 = Select(t=w319, s=w321, f="UP TO DATE") -> (s? t:f=w317:string)
                    n165 = local read "error out"() -> (w312:errorcluster)
                    n166 = local read "expired?"() -> (w330:bool)
                    n167 = local read "warn?"() -> (w331:bool)
                    n168 = Concatenate Strings(w326, w325, w343, w325, w327) -> (w328:string)
                    n169 = Select(t="EXPIRED", s=w340, f=w335) -> (s? t:f=w341:string)
                    n170 = local read "sn"() -> (w314:string)
                    n171 = Concatenate Strings(w339) -> (w338:string)
                    n172 = Build Array(w313, w314, w317, w316) -> (w315:string[])
                    n173 = Or(x=w331, y=w330) -> (x .or. y?=w329:bool)
                    n174 = Format Into String(format string=w333, error in=w312, w338, w328, w341, w342) -> (resulting string=w332:string, error out=w311:errorcluster)  [unwired: 1 in]
                  }
                }
              }
              n175 = Or Array Elements(Boolean array=w230) -> (logical OR=w225:bool)
              n176 = case shown="True" "Use Popup Warning(T)" {
                tunnel: w231 -> [_ w238]
                tunnel: w225 -> [_ w237]
                tunnel: w224 -> [w232 w236]
                tunnel: [w232 w234] -> w223
                frame False {
                }
                frame True {
                  n177 = case shown="True" w237 {
                    tunnel: w238 -> [_ w261]
                    tunnel: ["" w258] -> w239
                    tunnel: w236 -> [w251 w254]
                    tunnel: [w251 w254] -> w235
                    tunnel: [w250 w253] -> w233
                    frame False {
                      w250 = T1."Left Button"  # Which Button?
                    }
                    frame True {
                      w255 = "Open a copy of the cal record in excel"  # Right Button Text ("Cancel")
                      w256 = "Copy Message to Clipboard"  # Center Button Text ("No")
                      w257 = "Do Nothing ..Continue"  # Left Button Text ("Yes")
                      n178 = Array To Spreadsheet String(delimiter (Tab)="\r", array=w261, 3:"" ("format string")) -> (spreadsheet string=w258:string)
                      n179 = call <vilib>:"Three Button Dialog.vi"("Right Button Text (\"Cancel\")"=w255, "Center Button Text (\"No\")"=w256, "Left Button Text (\"Yes\")"=w257, "message"=w258) -> ("Which Button?"=w253:T1)  [unwired: 7 in]
                    }
                  }
                  n180 = case shown="\"Right Button\"" w233 {
                    tunnel: w239 -> [_ w243 _]
                    tunnel: w235 -> [w240 w242 w246]
                    tunnel: [w240 w241 w246] -> w234
                    frame "Left Button", Default {
                    }
                    frame "Center Button" {
                      n181 = invoke class="App" method="Clipboard.Write"(error in=w242, "Param 0"=w243) -> (error out=w241:errorcluster)  [unwired: 2 in, 3 out]
                    }
                    frame "Right Button" {
                      w248 = ","  # delimiter (\t)
                      n182 = disable-structure shown="Disabled" {
                        frame Disabled {
                          n183 = call <vilib>:"Generate Temporary File Path.vi"("Temporary File Extension (tmp)"="csv") -> ()  [unwired: 9 in, 2 out]
                        }
                        frame Enabled {
                        }
                      }
                      n184 = local read "RecordTempPath"() -> (w244:path)
                      n185 = local read "Record(ary)"() -> (w245:string[][])
                      n186 = call-poly <vilib>:"Write Delimited Spreadsheet.vi"("file path (dialog if empty)"=w244, "2D data"=w245, "delimiter (\\t)"=w248) -> ("new file path (Not A Path if cancelled)"=w247:path)  [unwired: 11 in, 1 out]
                      n187 = call "Open_Results_File_Excel.vi"("path to file"=w247) -> ()  [unwired: 10 in, 1 out]
                    }
                  }
                }
              }
              n188 = Not(x=w225) -> (.not. x?=w222:bool)
              n189 = Insert Into Array(array=w228, index (row)=0, new element=w227) -> (w221:string[][])  [unwired: 1 in]
            }
          }
        }
      }
    }
  }
  "Status Summary Out" <- w1
  n190 = local write "OK"(w2) -> ()
  n191 = local write "error out"(w4) -> ()
